vi "Set Limelight Pipeline.vi"(0 "Pipeline Number":dbl, 3 "error in":errorcluster) -> (10 "error out":errorcluster)   [LabVIEW 2019]
uses:
  <vilib>/Rock Robotics/Network Tables/NT Write Number.vi
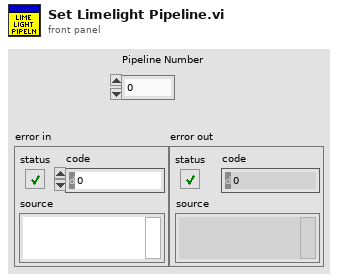
[diagram p1: front panel]
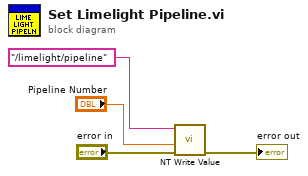
[diagram p0: block diagram]
diagram:
  n1 = call-poly <vilib>:"NT Write Value.vi"("error in"="error in", "Numeric"="Pipeline Number", "Name"="/limelight/pipeline") -> ("error out"=→"error out":errorcluster)  [unwired: 8 in]
